vi "Dual Servo Animation.vi"() -> ()   [LabVIEW 2023]
uses:
  <vilib>/LabVIEW Interface for Arduino/Type Defs/Board Type.ctl
  <vilib>/LabVIEW Interface for Arduino/Type Defs/Connection Type.ctl
  <vilib>/LabVIEW Interface for Arduino/LabVIEW Interface for Arduino.lvlib
panel:
  in  "Servo Number":u8=15
  in  "Servo Number 2":u8=15
  in  "DIO Pin (2) 2":u8=2
  in  "Servo Number (0) 2":u8
  out "Angle (Degrees) 2":u8=15
  in  "Angle (Degrees)":u8(knob)=15 scale=0.0..180.0
  in  "Servo Number":u8=15
  in  "stop":bool
  in  "DIO Pin (2)":u8=2
  in  "Servo Number (0)":u8
  in  "Number Of Servos (1)":u8=1
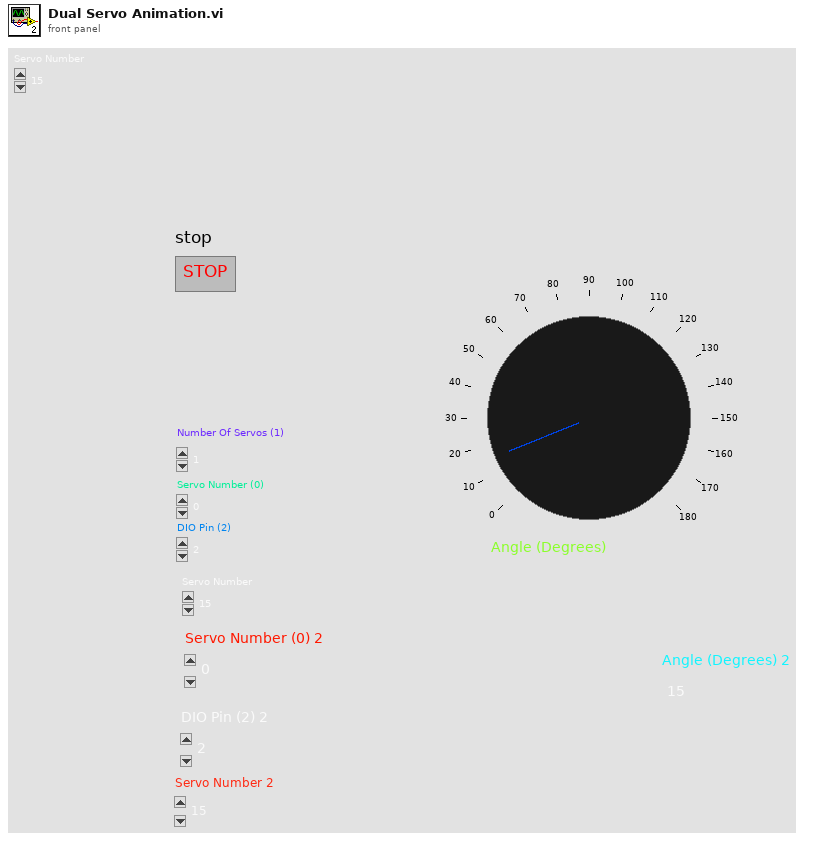
[diagram p1: front panel]
types:
  T1 = typedef "LabVIEW Interface for Arduino.lvlib/Connection Type.ctl" = enum8{"USB / Serial", "XBEE", "BlueSmirf (Bluetooth)"}
  T2 = typedef "LabVIEW Interface for Arduino.lvlib/Board Type.ctl" = enum16{"Uno", "Dimuelanove w/Atmega 328", "Mega 2560"}
  T3 = typedef "LabVIEW Interface for Arduino.lvlib/Arduino Resource.ctl" = cluster{"VISA resource":refnum<visa-resource-name>, "Board Type":T2, "Connection Type":enum8{"USB / Serial"}, "Bytes Per Packet (15)":u8}
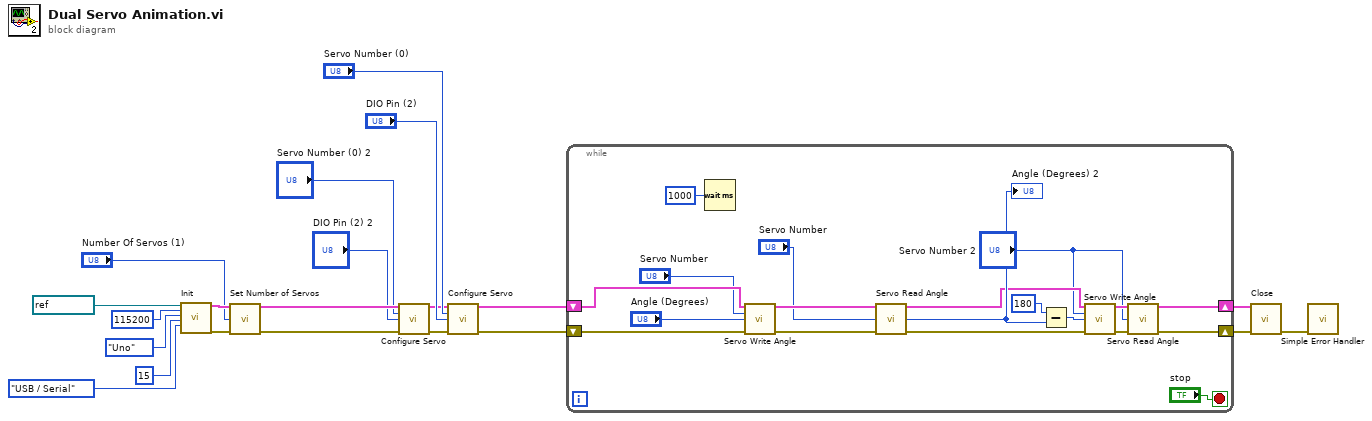
[diagram p0: block diagram]
diagram:
  n1 = call <vilib>:"Init.vi"("VISA resource"=refnum<visa-resource-name> "COM4", "Baud Rate (115200)"=u32 115200, "Board Type (Uno)"=Board_Type."Uno", "Bytes Per Packet (15)"=u32 15, "Connection Type (USB/Serial)"=Connection_Type."USB / Serial") -> ("Arduino Resource"=w21:T3, "error out"=w18:errorcluster)  [unwired: 13 in]
  n2 = call <vilib>:"Set Number of Servos.vi"("Arduino Resource"=w21, "Number Of Servos (1)"="Number Of Servos (1)", "error in"=w18) -> ("Arduino Resource"=w7:T3, "error out"=w5:errorcluster)  [unwired: 11 in]
  n3 = call <vilib>:"Configure Servo.vi"("Arduino Resource"=w7, "Servo Number (0)"="Servo Number (0) 2", "DIO Pin (2)"="DIO Pin (2) 2", "error in"=w5) -> ("Arduino Resource"=w6:T3, "error out"=w4:errorcluster)  [unwired: 10 in]
  n4 = call <vilib>:"Configure Servo.vi"("Arduino Resource"=w6, "Servo Number (0)"="Servo Number (0)", "DIO Pin (2)"="DIO Pin (2)", "error in"=w4) -> ("Arduino Resource"=w20:T3, "error out"=w17:errorcluster)  [unwired: 10 in]
  n5 = while {
    shift-right: [w29] -> w19
    shift-left: w20 -> [w40]
    shift-right: [w27] -> w16
    shift-left: w17 -> [w38]
    stop <- "stop" stop-if-true
    n6 = Wait (ms)(milliseconds to wait=u32 1000) -> ()  [unwired: 1 out]
    n7 = call <vilib>:"Servo Write Angle.vi"("Arduino Resource"=w40, "Servo Number"="Servo Number", "Angle (Degrees)"="Angle (Degrees)", "error in"=w38) -> ("Arduino Resource"=w39:T3, "error out"=w37:errorcluster)  [unwired: 10 in]
    n8 = call <vilib>:"Servo Read Angle.vi"("Arduino Resource"=w39, "Servo Number"="Servo Number", "error in"=w37) -> ("Arduino Resource"=w32:T3, "Angle (Degrees)"=w33:u8, "error out"=w31:errorcluster)  [unwired: 10 in]
    "Angle (Degrees) 2" <- w33
    n9 = Subtract(x=180, y=w33) -> (x-y=w30:i32)
    n10 = call <vilib>:"Servo Write Angle.vi"("Arduino Resource"=w32, "Servo Number"="Servo Number 2", "Angle (Degrees)"=w30, "error in"=w31) -> ("Arduino Resource"=w26:T3, "error out"=w28:errorcluster)  [unwired: 10 in]
    n11 = call <vilib>:"Servo Read Angle.vi"("Arduino Resource"=w26, "Servo Number"="Servo Number 2", "error in"=w28) -> ("Arduino Resource"=w29:T3, "error out"=w27:errorcluster)  [unwired: 10 in, 1 out]
  }
  n12 = call <vilib>:"Close.vi"("Arduino Resource"=w19, "error in"=w16) -> ("error out"=w1:errorcluster)  [unwired: 13 in]
  n13 = call <vilib>:"Simple Error Handler.vi"("error in (no error)"=w1) -> ()  [unwired: 4 in, 5 out]
